vi "Stop Core.vi"(10 "final error code":i32, 11 "Gui in":refnum<class "Gui.lvclass">) -> (3 "Gui out":refnum<class "Gui.lvclass">)   [LabVIEW 2022 SP3, in "Test.lvlib" / "Gui.lvlib" / "Gui.lvclass"]
doc: "(<B>Filename</B>: Actor Framework.lvlib:Actor.lvclass:Stop Core.vi)\n\nDefines what the actor does before it stops. Use the <B>final error code</B> input to determine whether the actor shut down in response to an error.\n\nBy default, this method does nothing. A descendant class may override it to define behavior, such as shutting down any processes the actor initiated in its override of the Actor Core method."
uses:
  Gui.lvclass
  Gui.lvclass/Gui.ctl
  LoggingActor/LoggingActor/LoggingActor.lvclass
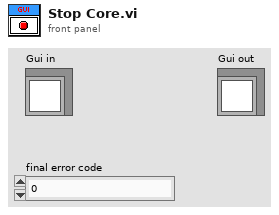
[diagram p1: front panel]
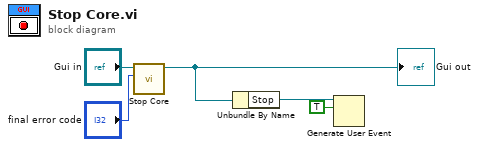
[diagram p0: block diagram]
diagram:
  n1 = call-parent "Stop Core.vi"("final error code"="final error code", "LoggingActor in"="Gui in") -> ("LoggingActor out"=w3:refnum<class "Gui.lvclass">)  [unwired: 9 in]
  "Gui out" <- w3
  n2 = Unbundle By Name(w3) -> ("Stop"=w2:refnum<user-event>)
  n3 = Generate User Event(user event=w2, event data cluster=TRUE ("event data")) -> ()  [unwired: 2 in, 2 out]
